vi "Raster.vi"(4 "Draw Lines":bool, 5 "Draw Triangles":bool, 6 "Line Colour":u32(colorbox)=4375295, 7 "Textured":bool, 10 "Triangles Sorted":T1[](array[typedef]) {"Vertex 3"."UV"."v" min=0 max=1 step=0.1; "Vertex 3"."UV"."u" min=0 max=1 step=0.1; "Vertex 2"."UV"."v" min=0 max=1 step=0.1; "Vertex 2"."UV"."u" min=0 max=1 step=0.1; "Vertex 1"."UV"."v" min=0 max=1 step=0.1; "Vertex 1"."UV"."u" min=0 max=1 step=0.1}, 11 "Pixel Data in":u32[][](array[numeric])) -> (3 "Pixel Data out":u32[][](array[numeric]))   [LabVIEW 2020, in "3D.lvlib"]
uses:
  3D.lvlib
  Raster/Raster.lvlib
  Raster/UV.ctl
  Raster/Rectangle Dimensions.ctl
  Raster/Texture.ctl
  Vector 3D.ctl
  Vertex.ctl
  Triangle.ctl
  Material.ctl
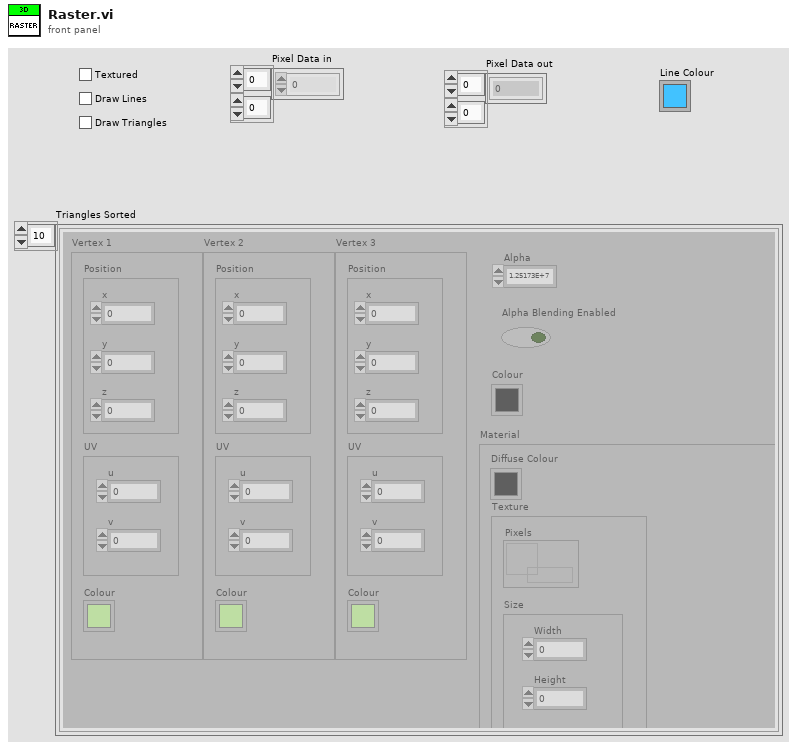
[diagram p1: front panel]
types:
  T1 = typedef "3D.lvlib/Triangle.ctl" = cluster{"Vertex 1":T2, "Vertex 2":T2, "Vertex 3":T2, "Alpha":dbl, "Alpha Blending Enabled":bool, "Colour":u32, "Material":T5}
  T2 = typedef "3D.lvlib/Vertex.ctl" = cluster{"Position":T3, "UV":T4, "Colour":u32}
  T3 = typedef "3D.lvlib/Vector 3D.ctl" = cluster{"x":sgl, "y":sgl, "z":sgl}
  T4 = typedef "Raster.lvlib/UV.ctl" = cluster{"u":sgl, "v":sgl}
  T5 = typedef "3D.lvlib/Material.ctl" = cluster{"Diffuse Colour":u32, "Texture":T6}
  T6 = typedef "Raster.lvlib/Texture.ctl" = cluster{"Pixels":refnum<data-value>, "Size":T7}
  T7 = typedef "Raster.lvlib/Rectangle Dimensions.ctl" = cluster{"Width":u32, "Height":u32}
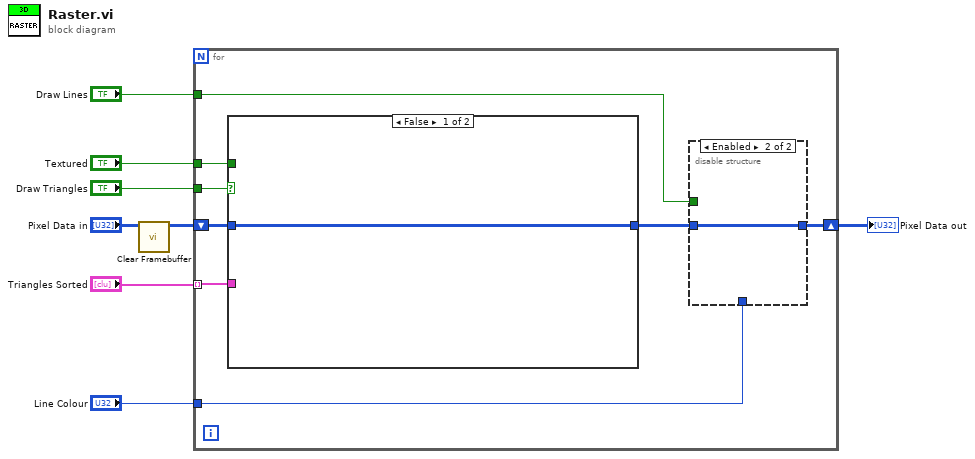
[diagram p0: block diagram]
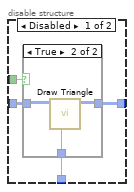
[diagram p2: hidden frame]
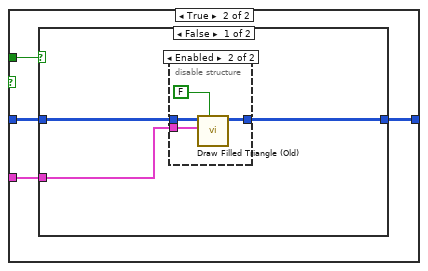
[diagram p4: hidden frame]
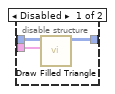
[diagram p5: hidden frame]
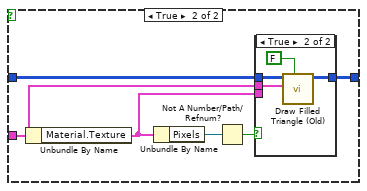
[diagram p6: hidden frame]
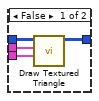
[diagram p7: hidden frame]
diagram:
  n1 = call "Clear Framebuffer.vi"("Pixel Data in"="Pixel Data in") -> ("Pixel Data out"=w4:u32[][])  [unwired: 10 in]
  n2 = for {
    tunnel: "Line Colour" -> [w16]
    tunnel: "Triangles Sorted" -> [w10] mode=indexing
    tunnel: "Draw Lines" -> [w15]
    tunnel: "Draw Triangles" -> [w12]
    shift-right: [w11] -> w2
    shift-left: w4 -> [w14]
    tunnel: "Textured" -> [w9]
    n3 = case shown="False" w12 {
      tunnel: w14 -> [w26 w30]
      tunnel: [w26 w29] -> w13
      tunnel: w10 -> [_ w28]
      tunnel: w9 -> [_ w27]
      frame False {
      }
      frame True {
        n4 = case shown="False" w27 {
          tunnel: w30 -> [w33 w46]
          tunnel: [w32 w45] -> w29
          tunnel: w28 -> [w31 w44]
          frame False {
            n5 = disable-structure shown="Enabled" {
              disable-tunnel: w33 -> [w36 w40]
              disable-tunnel: [w35 w39] -> w32
              disable-tunnel: w31 -> [w34 w38]
              frame Disabled {
                n6 = call "Draw Filled Triangle.vi"("Triangle"=w34, "Pixel Data in"=w36) -> ("Pixel Data out"=w35:u32[][])  [unwired: 9 in]
              }
              frame Enabled {
                n7 = call "Draw Filled Triangle (Old).vi"("Enable Alpha Blending (F)"=FALSE, "Triangle"=w38, "Pixel Data in"=w40) -> ("Pixel Data out"=w39:u32[][])  [unwired: 8 in]
              }
            }
          }
          frame True {
            n8 = Unbundle By Name(w44) -> ("Material.Texture"=w43:T6)
            n9 = Unbundle By Name(w43) -> ("Pixels"=w42:refnum<data-value>)
            n10 = Not A Number/Path/Refnum?(number/path/refnum=w42) -> (NaN/Path/Refnum?=w41:bool)
            n11 = case shown="True" w41 {
              tunnel: w46 -> [w50 w53]
              tunnel: [w49 w52] -> w45
              tunnel: w44 -> [w48 w51]
              tunnel: w43 -> [w47 _]
              frame False {
                n12 = call "Draw Textured Triangle.vi"("Texture"=w47, "Triangle"=w48, "Pixel Data in"=w50) -> ("Pixel Data out"=w49:u32[][])  [unwired: 8 in]
              }
              frame True {
                n13 = call "Draw Filled Triangle (Old).vi"("Enable Alpha Blending (F)"=FALSE, "Triangle"=w51, "Pixel Data in"=w53) -> ("Pixel Data out"=w52:u32[][])  [unwired: 8 in]
              }
            }
          }
        }
      }
    }
    n14 = disable-structure shown="Enabled" {
      disable-tunnel: w16 -> [w20 _]
      disable-tunnel: w15 -> [w19 _]
      disable-tunnel: w13 -> [w18 w25]
      disable-tunnel: [w17 w25] -> w11
      frame Disabled {
        n15 = case shown="True" w19 {
          tunnel: w18 -> [w21 w23]
          tunnel: w20 -> [_ w24]
          tunnel: [w21 w22] -> w17
          frame False {
          }
          frame True {
            n16 = call "Draw Triangle.vi"("Line Colour"=w24, "Pixel Data in"=w23) -> ("Pixel Data out"=w22:u32[][])  [unwired: 9 in]
          }
        }
      }
      frame Enabled {
      }
    }
  }
  "Pixel Data out" <- w2
